vi "Target - Async (Reentrant).vi"(9 "Wait (Milliseconds)":u32, 10 "Y":dbl, 11 "X":dbl) -> (3 "X + Y":dbl)   [LabVIEW 2016]
doc: "Target VI used with the asynchronous call examples. This VI is reentrant."
panel:
  out "Time Remaining (Seconds)":dbl format="%#.1f"
  # "Target VI used with the asynchronous call examples. This VI is reentrant."
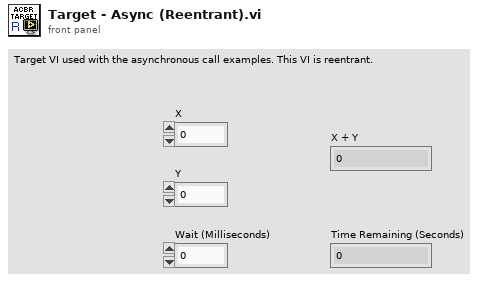
[diagram p1: front panel]
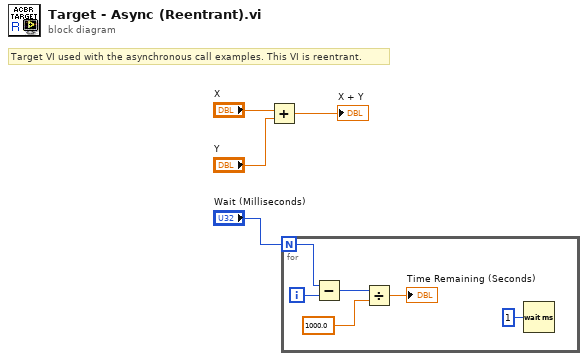
[diagram p0: block diagram]
diagram:
  # "Target VI used with the asynchronous call examples. This VI is reentrant."
  n1 = Add(x="X", y="Y") -> (x+y=→"X + Y":dbl)
  n2 = for {
    N: "Wait (Milliseconds)" -> [w9]
    i -> [w8]
    n3 = Subtract(x=w9, y=w8) -> (x-y=w7:i32)
    n4 = Divide(x=w7, y=1000.0) -> (x/y=→"Time Remaining (Seconds)":dbl)
    n5 = Wait (ms)(milliseconds to wait=u32 1) -> ()  [unwired: 1 out]
  }
